vi "PID_controller_11.vi"() -> ()   [LabVIEW 2011]
uses:
  <vilib>/Platform/TimedLoop/XDataNode/timing_clust.ctl
  <vilib>/Platform/TimedLoop/XDataNode/nitl_modes.ctl
  <vilib>/Platform/TimedLoop/XDataNode/wakeup.ctl
  <vilib>/Platform/TimedLoop/XDataNode/XDataNode.xnode
  <vilib>/Platform/TimedLoop/XDataNode/XDNodeRunTimeDep.lvlib
panel:
  in  "stop 2":bool
  out "fit":cluster{"element":dbl, "Value":dbl}[](array[cluster])
  out "err_avg":dbl
  out "Setpoint":string
  out "Angle (deg)":string
  in  "Ks":dbl
  out "dt(s)":dbl
  out "windup error":dbl
  out "tPrev":dbl
  out "target value":dbl
  out "error(t-t0)":cluster{dbl, "Value":dbl}[](array[cluster])
  out "error":dbl
  out "tStart(s)":dbl
  out "S00":dbl
  out "S10":dbl
  out "S20":dbl
  out "S11":dbl
  out "S01":dbl
  out "weight":dbl[](array[numeric])
  in  "# of points to watch":i32
  in  "tSmooth(s)":dbl=-1.0
  out "t0":dbl
  out "error(t)":cluster{dbl, "Value":dbl}[](array[cluster])
  out "error out":errorcluster
  out "first":bool=TRUE
  out "P (torr)":string
  out "XY Graph":T1(graph)
  out "current value":dbl
  in  "Period (s)":dbl
  out "dValue":dbl
  out "derivative":dbl
  out "integral":dbl
  out "Current angle (deg)":dbl
  in  "Kd":dbl
  in  "Ki":dbl
  in  "Kp":dbl
  out "Current P (torr)":dbl
  in  "Set Point (torr)":dbl
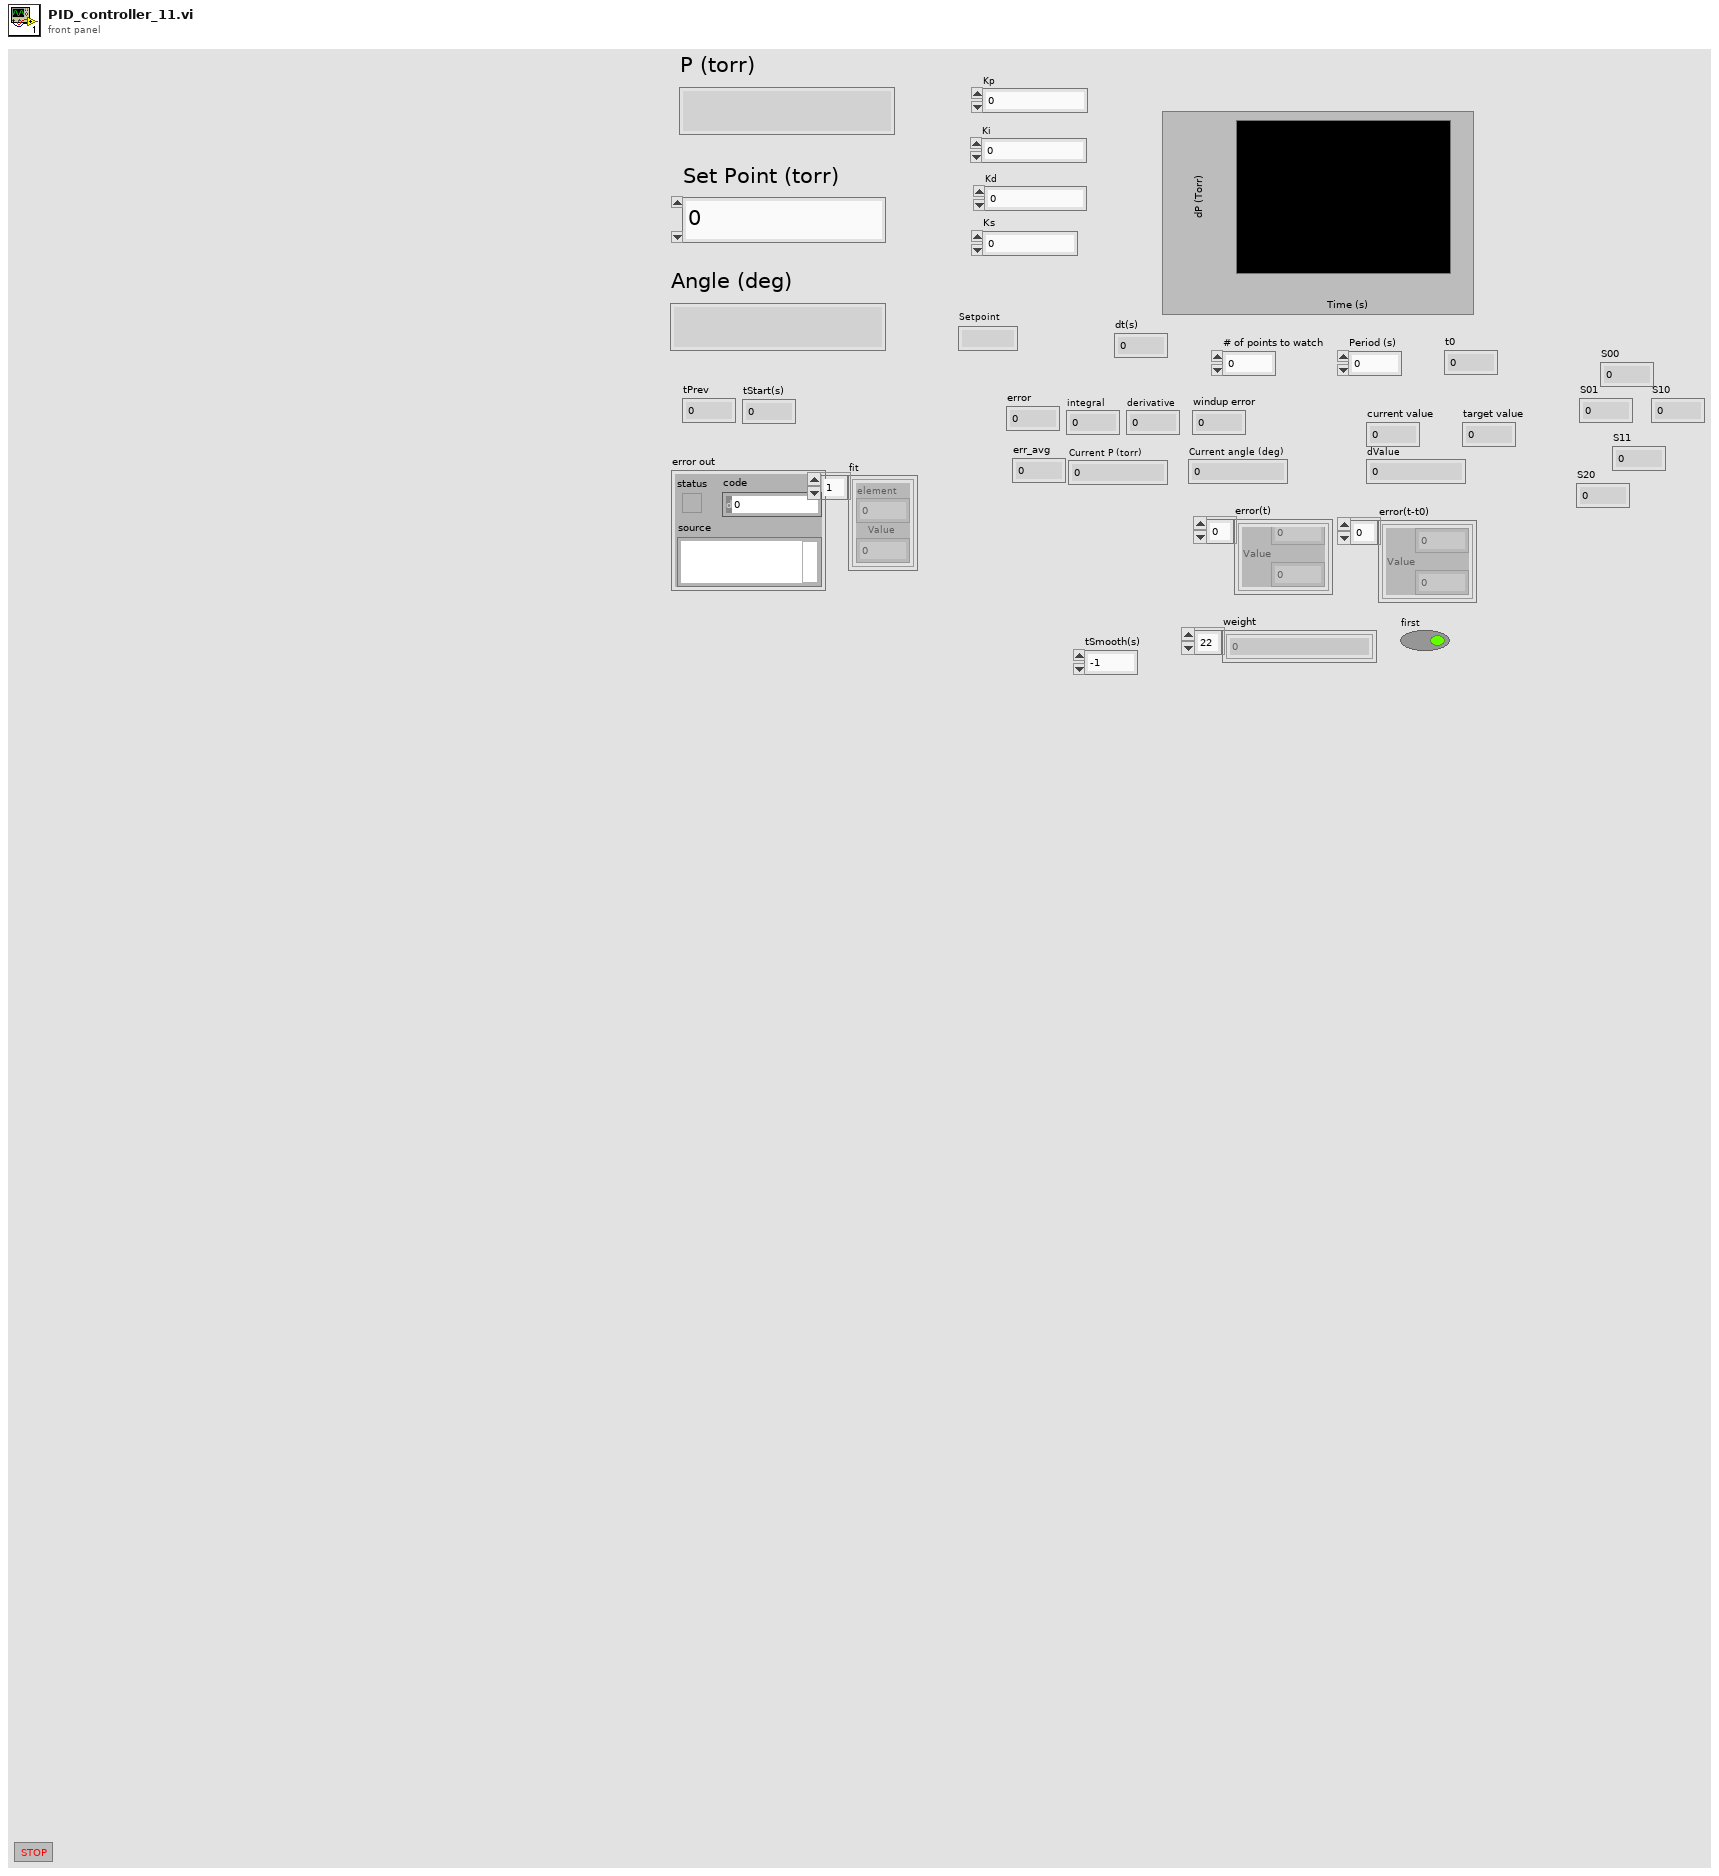
[diagram p1: front panel]
types:
  T1 = cluster{"Value":cluster{"element":dbl, "Value":dbl}[]}[]
  T2 = typedef "XDNodeRunTimeDep.lvlib/timing_clust.ctl" = cluster{"Expected End [f-1]":u64, "Actual End [f-1]":u64, "Finished Late? [f-1]":bool, "Expected End [i-1]":u64, "Actual End [i-1]":u64, "Finished Late? [i-1]":bool, "Expected Start [i]":u64, "Actual Start [i]":u64, "Expected Start [f]":u64, "Actual Start [f]":u64, "Source Name":string, "Structure Name":string, "Period":i64, "Deadline":i64, "Offset":i64, "Start":i64, "Priority":i32, "Timeout":i32, "Mode":T3, "Wakeup Reason":T4, "Error":errorcluster, "Source Type":string, "Secondary Source Type":string, "Global End Time":u64, "Global Start Time":u64, "Frame Duration":u64, "Iteration Duration":u64, "Assigned CPU":i32, "I/O Scan Engine Mode":u32}
  T3 = typedef "XDNodeRunTimeDep.lvlib/nitl_modes.ctl" = enum32{"No Change", "Process missed periods, maintain original phase", "Discard missed periods, maintain original phase", "Process missed periods, ignore original phase", "Discard missed periods, ignore original phase"}
  T4 = typedef "XDNodeRunTimeDep.lvlib/wakeup.ctl" = enum32{"Normal", "Aborted", "Asynchronous wakeup", "Timing source error", "Timed loop error", "Timeout"}
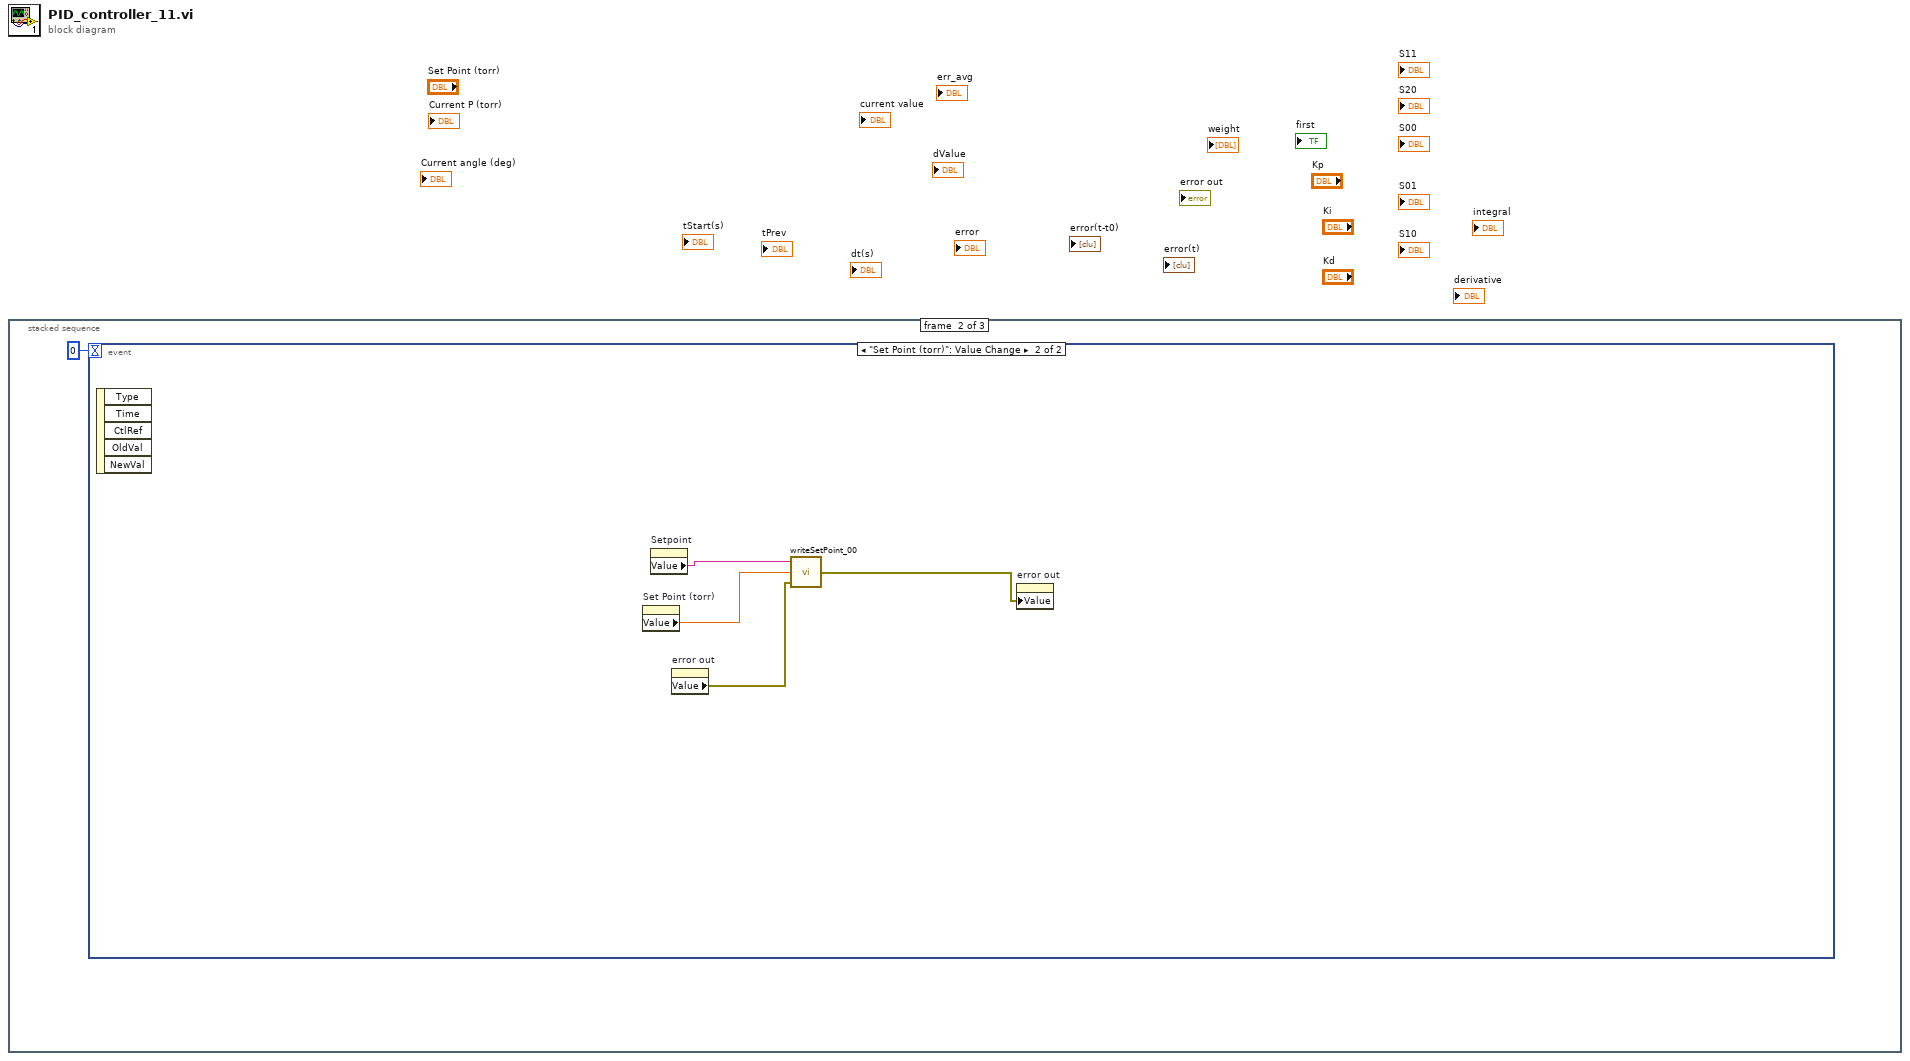
[diagram p0: block diagram]
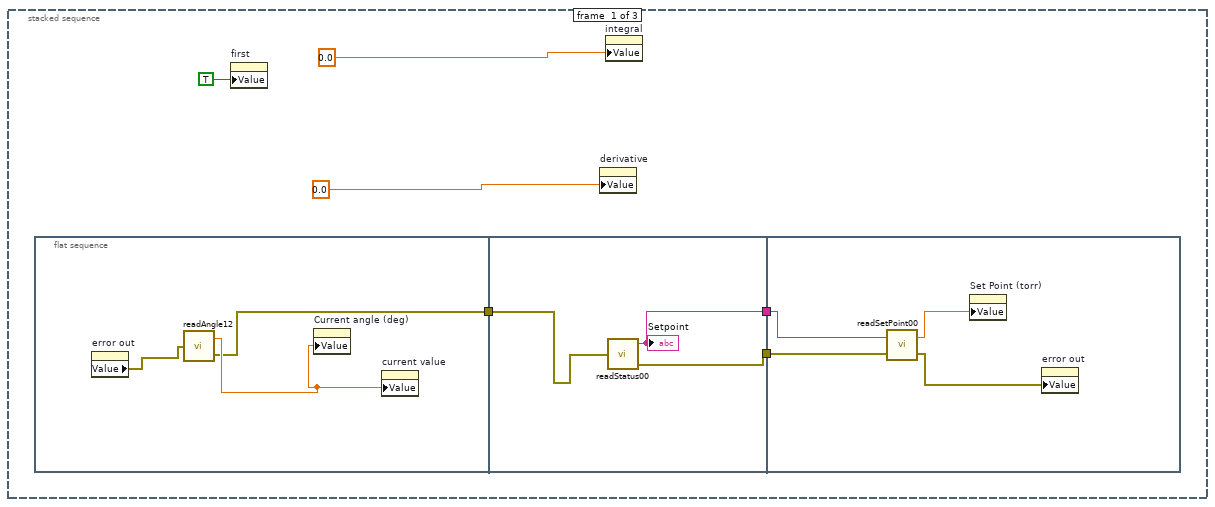
[diagram p2: hidden frame]
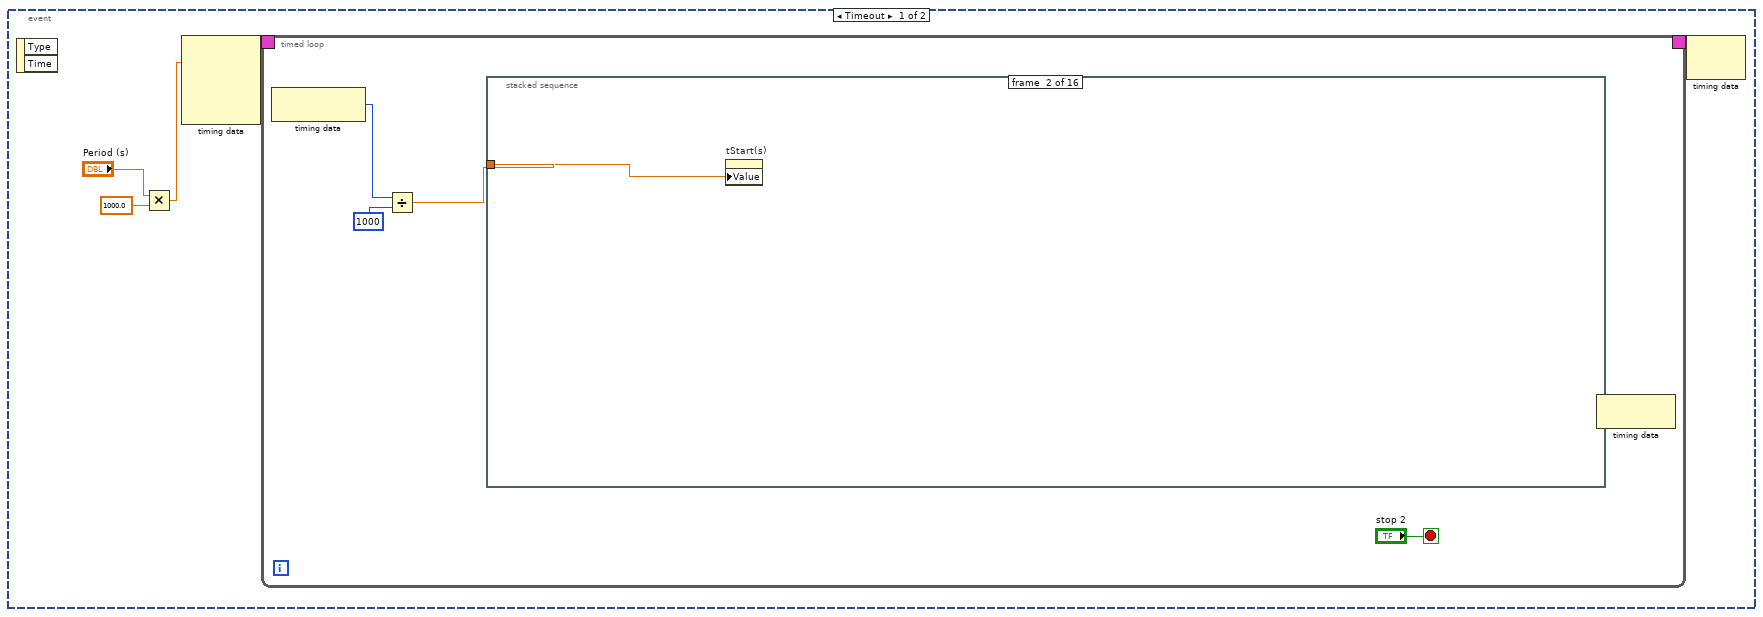
[diagram p3: hidden frame]
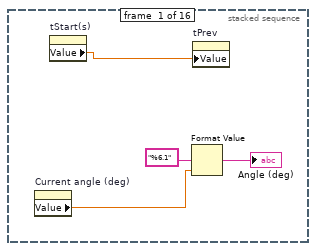
[diagram p4: hidden frame]
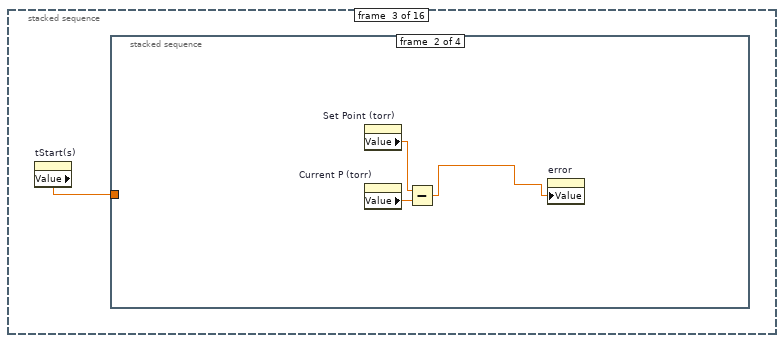
[diagram p5: hidden frame]
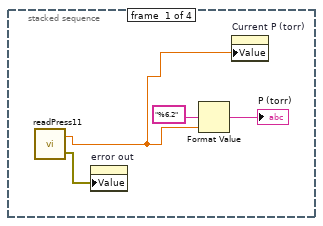
[diagram p6: hidden frame]
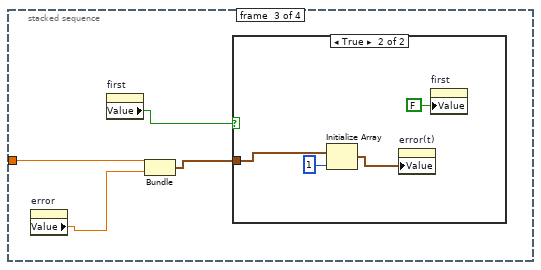
[diagram p7: hidden frame]
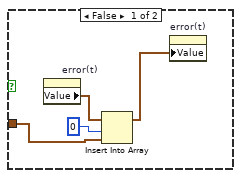
[diagram p8: hidden frame]
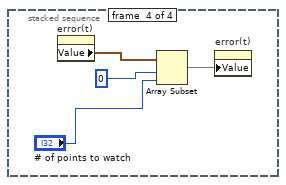
[diagram p9: hidden frame]
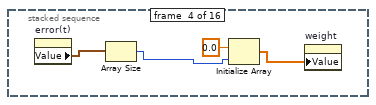
[diagram p10: hidden frame]
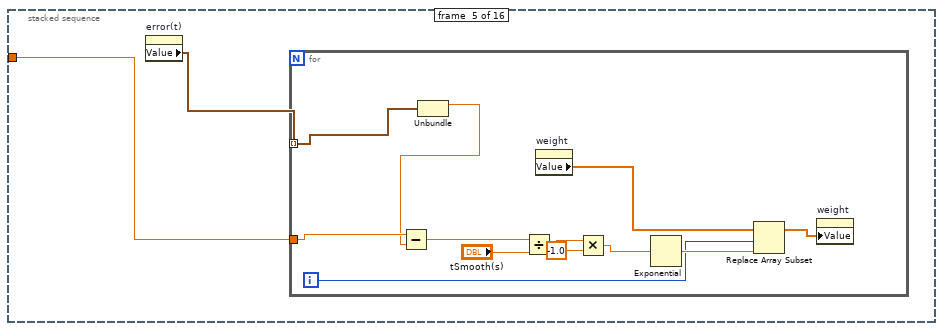
[diagram p11: hidden frame]
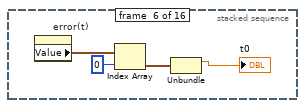
[diagram p12: hidden frame]
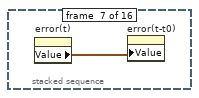
[diagram p13: hidden frame]
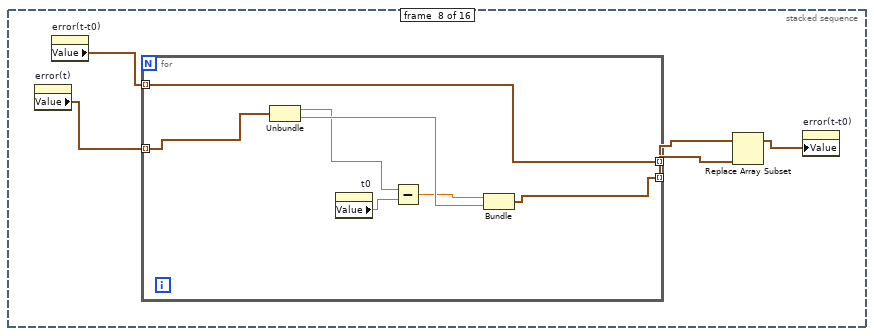
[diagram p14: hidden frame]
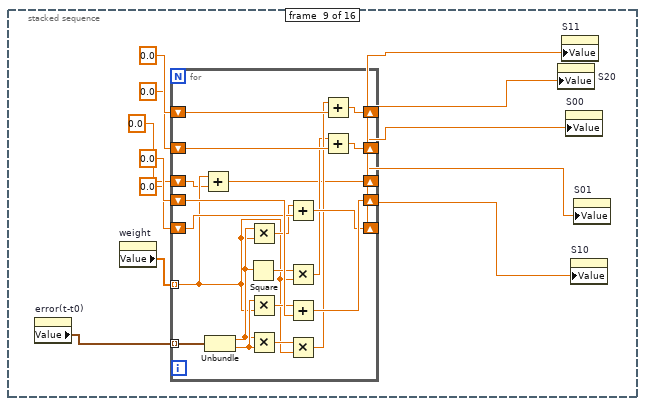
[diagram p15: hidden frame]
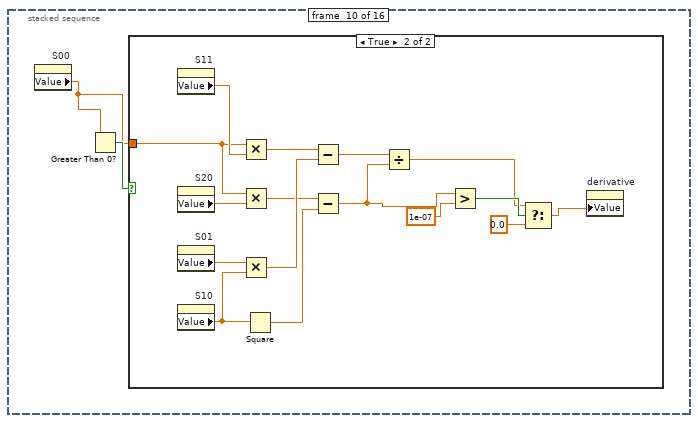
[diagram p16: hidden frame]
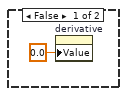
[diagram p17: hidden frame]
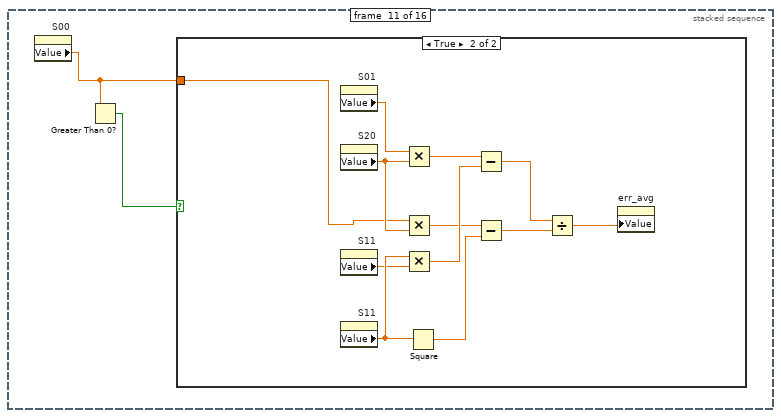
[diagram p18: hidden frame]
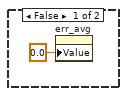
[diagram p19: hidden frame]
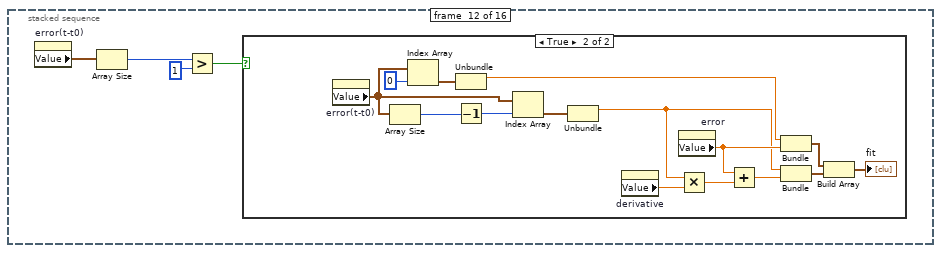
[diagram p20: hidden frame]
diagram:
  n1 = stacked-sequence {
    frame #0 {
      n2 = flat-sequence {
        tunnel: [w7] -> w1
        tunnel: [w12] -> w3
        tunnel: [w11] -> w2
        tunnel: w1 -> [w10]
        tunnel: w3 -> [w16]
        tunnel: w2 -> [w15]
        frame #0 {
          n3 = property on="error out" class="Clust (strict)"() -> ("Value"=w9:errorcluster)  [unwired: 2 in, 2 out]
          n4 = call "readAngle12.vi"("error in"=w9) -> ("angle"=w8:dbl, "error out"=w7:errorcluster)
          n5 = property on="Current angle (deg)" class="DigNum (strict)"("Value"=w8) -> ()  [unwired: 2 in, 2 out]
          n6 = property on="current value" class="DigNum (strict)"("Value"=w8) -> ()  [unwired: 2 in, 2 out]
        }
        frame #1 {
          n7 = call "readStatus00.vi"("error in"=w10) -> ("Setpoint"=w12:string, "error out"=w11:errorcluster)  [unwired: 1 out]
          "Setpoint" <- w12
        }
        frame #2 {
          n8 = call "readSetPoint00.vi"("error in"=w15, "Setpoint"=w16) -> ("error out"=w14:errorcluster, "P"=w13:dbl)
          n9 = property on="Set Point (torr)" class="DigNum (strict)"("Value"=w13) -> ()  [unwired: 2 in, 2 out]
          n10 = property on="error out" class="Clust (strict)"("Value"=w14) -> ()  [unwired: 2 in, 2 out]
        }
      }
      n11 = property on="first" class="Bool (strict)"("Value"=TRUE ("first")) -> ()  [unwired: 2 in, 2 out]
      n12 = property on="derivative" class="DigNum (strict)"("Value"=0.0 ("derivative")) -> ()  [unwired: 2 in, 2 out]
      n13 = property on="integral" class="DigNum (strict)"("Value"=0.0 ("integral")) -> ()  [unwired: 2 in, 2 out]
    }
    frame #1 {
      n14 = event shown="[1] \"Set Point (torr)\": Value Change" {
        selector: _ -> [_ _]
        dyn-events: _ -> [_ _]
        timeout: 0 -> [_ _]
        event Timeout {
          n15 = event-data() -> ()  [unwired: 1 in, 2 out]
          n16 = Multiply(x="Period (s)", y=1000.0) -> (x*y=w18:dbl)
          n17 = node-c288(w18) -> (w22:T2)  [unwired: 3 in]
          n18 = timed-loop {
            timing: w22 -> [_]
            timing-out: [_] -> w21
            stop <- "stop 2" stop-if-true
            n19 = node-c288() -> (w24:i64)  [unwired: 1 in]
            n20 = Divide(x=w24, y=i64 1000) -> (x/y=w23:dbl)
            n21 = stacked-sequence {
              tunnel: w23 -> [_ w31 _ _ w60 _ _ _ _ _ _ _ _ _ _ _]
              frame #0 {
                n22 = property on="Current angle (deg)" class="DigNum (strict)"() -> ("Value"=w27:dbl)  [unwired: 2 in, 2 out]
                n23 = property on="tStart(s)" class="DigNum (strict)"() -> ("Value"=w30:dbl)  [unwired: 2 in, 2 out]
                n24 = Format Value(format string="%6.1", value (0)=w27) -> (output string=→"Angle (deg)":string)  [unwired: 1 in]
                n25 = property on="tPrev" class="DigNum (strict)"("Value"=w30) -> ()  [unwired: 2 in, 2 out]
              }
              frame #1 {
                n26 = property on="tStart(s)" class="DigNum (strict)"("Value"=w31) -> ()  [unwired: 2 in, 2 out]
              }
              frame #2 {
                n27 = property on="tStart(s)" class="DigNum (strict)"() -> ("Value"=w32:dbl)  [unwired: 2 in, 2 out]
                n28 = stacked-sequence {
                  tunnel: w32 -> [_ _ w42 _]
                  frame #0 {
                    n29 = call "readPress11.vi"() -> ("P"=w34:dbl, "error out"=w33:errorcluster)  [unwired: 1 in]
                    n30 = property on="error out" class="Clust (strict)"("Value"=w33) -> ()  [unwired: 2 in, 2 out]
                    n31 = Format Value(format string="%6.2", value (0)=w34) -> (output string=→"P (torr)":string)  [unwired: 1 in]
                    n32 = property on="Current P (torr)" class="DigNum (strict)"("Value"=w34) -> ()  [unwired: 2 in, 2 out]
                  }
                  frame #1 {
                    n33 = property on="Set Point (torr)" class="DigNum (strict)"() -> ("Value"=w38:dbl)  [unwired: 2 in, 2 out]
                    n34 = property on="Current P (torr)" class="DigNum (strict)"() -> ("Value"=w39:dbl)  [unwired: 2 in, 2 out]
                    n35 = Subtract(x=w38, y=w39) -> (x-y=w37:dbl)
                    n36 = property on="error" class="DigNum (strict)"("Value"=w37) -> ()  [unwired: 2 in, 2 out]
                  }
                  frame #2 {
                    n37 = property on="error" class="DigNum (strict)"() -> ("Value"=w40:dbl)  [unwired: 2 in, 2 out]
                    n38 = property on="first" class="Bool (strict)"() -> ("Value"=w43:bool)  [unwired: 2 in, 2 out]
                    n39 = Bundle("Value"=w42, "Value"=w40) -> (w41:cluster{"Value":dbl, "Value":dbl})  [unwired: 1 in]
                    n40 = case shown="True" w43 {
                      tunnel: w41 -> [w45 w50]
                      frame False {
                        n41 = property on="error(t)" class="Arr (strict)"() -> ("Value"=w46:cluster{dbl, "Value":dbl}[])  [unwired: 2 in, 2 out]
                        n42 = Insert Into Array(array=w46, index=0, new element=w45) -> (w44:cluster{dbl, "Value":dbl}[])
                        n43 = property on="error(t)" class="Arr (strict)"("Value"=w44) -> ()  [unwired: 2 in, 2 out]
                      }
                      frame True {
                        n44 = Initialize Array(w50, 1 ("dimension size")) -> (w48:cluster{"Value":dbl, "Value":dbl}[])
                        n45 = property on="error(t)" class="Arr (strict)"("Value"=w48) -> ()  [unwired: 2 in, 2 out]
                        n46 = property on="first" class="Bool (strict)"("Value"=FALSE ("first")) -> ()  [unwired: 2 in, 2 out]
                      }
                    }
                  }
                  frame #3 {
                    n47 = property on="error(t)" class="Arr (strict)"() -> ("Value"=w53:cluster{dbl, "Value":dbl}[])  [unwired: 2 in, 2 out]
                    n48 = Array Subset(array=w53, index=0, length="# of points to watch") -> (w55:cluster{dbl, "Value":dbl}[])
                    n49 = property on="error(t)" class="Arr (strict)"("Value"=w55) -> ()  [unwired: 2 in, 2 out]
                  }
                }
              }
              frame #3 {
                n50 = property on="error(t)" class="Arr (strict)"() -> ("Value"=w59:cluster{dbl, "Value":dbl}[])  [unwired: 2 in, 2 out]
                n51 = Array Size(array=w59) -> (size(s)=w57:i32)
                n52 = Initialize Array(0.0 ("element"), w57) -> (w56:dbl[])
                n53 = property on="weight" class="Arr (strict)"("Value"=w56) -> ()  [unwired: 2 in, 2 out]
              }
              frame #4 {
                n54 = property on="error(t)" class="Arr (strict)"() -> ("Value"=w61:cluster{dbl, "Value":dbl}[])  [unwired: 2 in, 2 out]
                n55 = for {
                  tunnel: w61 -> [w73] mode=indexing
                  tunnel: w60 -> [w72]
                  i -> [w68]
                  n56 = Unbundle(w73) -> (w71:dbl)  [unwired: 1 out]
                  n57 = Subtract(x=w72, y=w71) -> (x-y=w66:dbl)
                  n58 = Divide(x=w66, y="tSmooth(s)") -> (x/y=w64:dbl)
                  n59 = property on="weight" class="Arr (strict)"() -> ("Value"=w69:dbl[])  [unwired: 2 in, 2 out]
                  n60 = Multiply(x=w64, y=-1.0) -> (x*y=w62:dbl)
                  n61 = Exponential(1:w62) -> (0:w70:dbl)
                  n62 = Replace Array Subset(array=w69, new element=w70, index=w68) -> (w67:dbl[])
                  n63 = property on="weight" class="Arr (strict)"("Value"=w67) -> ()  [unwired: 2 in, 2 out]
                }
              }
              frame #5 {
                n64 = property on="error(t)" class="Arr (strict)"() -> ("Value"=w77:cluster{dbl, "Value":dbl}[])  [unwired: 2 in, 2 out]
                n65 = Index Array(array=w77, index=0) -> (element=w75:cluster{dbl, "Value":dbl})
                n66 = Unbundle(w75) -> (→"t0":dbl)  [unwired: 1 out]
              }
              frame #6 {
                n67 = property on="error(t)" class="Arr (strict)"() -> ("Value"=w78:cluster{dbl, "Value":dbl}[])  [unwired: 2 in, 2 out]
                n68 = property on="error(t-t0)" class="Arr (strict)"("Value"=w78) -> ()  [unwired: 2 in, 2 out]
              }
              frame #7 {
                n69 = property on="error(t)" class="Arr (strict)"() -> ("Value"=w83:cluster{dbl, "Value":dbl}[])  [unwired: 2 in, 2 out]
                n70 = property on="error(t-t0)" class="Arr (strict)"() -> ("Value"=w81:cluster{dbl, "Value":dbl}[])  [unwired: 2 in, 2 out]
                n71 = for {
                  tunnel: w83 -> [w86] mode=indexing
                  tunnel: [w85] -> w82 mode=indexing
                  tunnel: w81 -> [w84] mode=indexing
                  tunnel: [w84] -> w80 mode=indexing
                  n72 = Unbundle(w86) -> (w87:dbl, "Value"=w89:dbl)
                  n73 = property on="t0" class="DigNum (strict)"() -> ("Value"=w90:dbl)  [unwired: 2 in, 2 out]
                  n74 = Subtract(x=w87, y=w90) -> (x-y=w88:dbl)
                  n75 = Bundle(w88, "Value"=w89) -> (w85:cluster{dbl, "Value":dbl})  [unwired: 1 in]
                }
                n76 = Replace Array Subset(array=w80, new element=w82) -> (w79:cluster{dbl, "Value":dbl}[])  [unwired: 1 in]
                n77 = property on="error(t-t0)" class="Arr (strict)"("Value"=w79) -> ()  [unwired: 2 in, 2 out]
              }
              frame #8 {
                n78 = property on="error(t-t0)" class="Arr (strict)"() -> ("Value"=w91:cluster{dbl, "Value":dbl}[])  [unwired: 2 in, 2 out]
                n79 = property on="weight" class="Arr (strict)"() -> ("Value"=w98:dbl[])  [unwired: 2 in, 2 out]
                n80 = for {
                  tunnel: w91 -> [w118] mode=indexing
                  shift-right: [w119] -> w93
                  shift-left: 0.0 -> [w122]
                  shift-right: [w115] -> w96
                  shift-left: 0.0 -> [w121]
                  shift-right: [w114] -> w95
                  shift-left: 0.0 -> [w120]
                  shift-right: [w116] -> w92
                  shift-left: 0.0 -> [w117]
                  tunnel: w98 -> [w105] mode=indexing
                  shift-right: [w103] -> w94
                  shift-left: 0.0 -> [w104]
                  n81 = Add(x=w105, y=w104) -> (x+y=w103:dbl)
                  n82 = Unbundle(w118) -> (w107:dbl, "Value"=w113:dbl)
                  n83 = Square(x=w107) -> (x^2=w109:dbl)
                  n84 = Multiply(x=w107, y=w105) -> (x*y=w106:dbl)
                  n85 = Multiply(x=w113, y=w105) -> (x*y=w112:dbl)
                  n86 = Multiply(x=w107, y=w113) -> (x*y=w111:dbl)
                  n87 = Add(x=w106, y=w117) -> (x+y=w116:dbl)
                  n88 = Multiply(x=w109, y=w105) -> (x*y=w108:dbl)
                  n89 = Add(x=w112, y=w122) -> (x+y=w119:dbl)
                  n90 = Multiply(x=w111, y=w105) -> (x*y=w110:dbl)
                  n91 = Add(x=w110, y=w121) -> (x+y=w115:dbl)
                  n92 = Add(x=w108, y=w120) -> (x+y=w114:dbl)
                }
                n93 = property on="S20" class="DigNum (strict)"("Value"=w95) -> ()  [unwired: 2 in, 2 out]
                n94 = property on="S11" class="DigNum (strict)"("Value"=w96) -> ()  [unwired: 2 in, 2 out]
                n95 = property on="S00" class="DigNum (strict)"("Value"=w94) -> ()  [unwired: 2 in, 2 out]
                n96 = property on="S10" class="DigNum (strict)"("Value"=w92) -> ()  [unwired: 2 in, 2 out]
                n97 = property on="S01" class="DigNum (strict)"("Value"=w93) -> ()  [unwired: 2 in, 2 out]
              }
              frame #9 {
                n98 = property on="S00" class="DigNum (strict)"() -> ("Value"=w123:dbl)  [unwired: 2 in, 2 out]
                n99 = Greater Than 0?(x=w123) -> (x > 0?=w124:bool)
                n100 = case shown="True" w124 {
                  tunnel: w123 -> [_ w133]
                  frame False {
                    n101 = property on="derivative" class="DigNum (strict)"("Value"=0.0 ("derivative")) -> ()  [unwired: 2 in, 2 out]
                  }
                  frame True {
                    n102 = property on="S11" class="DigNum (strict)"() -> ("Value"=w135:dbl)  [unwired: 2 in, 2 out]
                    n103 = property on="S20" class="DigNum (strict)"() -> ("Value"=w134:dbl)  [unwired: 2 in, 2 out]
                    n104 = property on="S01" class="DigNum (strict)"() -> ("Value"=w132:dbl)  [unwired: 2 in, 2 out]
                    n105 = property on="S10" class="DigNum (strict)"() -> ("Value"=w136:dbl)  [unwired: 2 in, 2 out]
                    n106 = Multiply(x=w133, y=w135) -> (x*y=w141:dbl)
                    n107 = Multiply(x=w133, y=w134) -> (x*y=w139:dbl)
                    n108 = Multiply(x=w132, y=w136) -> (x*y=w140:dbl)
                    n109 = Square(x=w136) -> (x^2=w138:dbl)
                    n110 = Subtract(x=w141, y=w140) -> (x-y=w137:dbl)
                    n111 = Subtract(x=w139, y=w138) -> (x-y=w131:dbl)
                    n112 = Divide(x=w137, y=w131) -> (x/y=w127:dbl)
                    n113 = Greater?(x=w131, y=1e-07) -> (0:w129:bool)
                    n114 = Select(t=w127, s=w129, f=0.0) -> (s? t:f=w128:dbl)
                    n115 = property on="derivative" class="DigNum (strict)"("Value"=w128) -> ()  [unwired: 2 in, 2 out]
                  }
                }
              }
              frame #10 {
                n116 = property on="S00" class="DigNum (strict)"() -> ("Value"=w142:dbl)  [unwired: 2 in, 2 out]
                n117 = Greater Than 0?(x=w142) -> (x > 0?=w143:bool)
                n118 = case shown="True" w143 {
                  tunnel: w142 -> [_ w146]
                  frame False {
                    n119 = property on="err_avg" class="DigNum (strict)"("Value"=0.0 ("Pavg")) -> ()  [unwired: 2 in, 2 out]
                  }
                  frame True {
                    n120 = property on="S01" class="DigNum (strict)"() -> ("Value"=w147:dbl)  [unwired: 2 in, 2 out]
                    n121 = property on="S20" class="DigNum (strict)"() -> ("Value"=w150:dbl)  [unwired: 2 in, 2 out]
                    n122 = property on="S11" class="DigNum (strict)"() -> ("Value"=w148:dbl)  [unwired: 2 in, 2 out]
                    n123 = property on="S11" class="DigNum (strict)"() -> ("Value"=w149:dbl)  [unwired: 2 in, 2 out]
                    n124 = Multiply(x=w147, y=w150) -> (x*y=w155:dbl)
                    n125 = Multiply(x=w146, y=w150) -> (x*y=w152:dbl)
                    n126 = Multiply(x=w149, y=w148) -> (x*y=w156:dbl)
                    n127 = Square(x=w149) -> (x^2=w153:dbl)
                    n128 = Subtract(x=w155, y=w156) -> (x-y=w151:dbl)
                    n129 = Subtract(x=w152, y=w153) -> (x-y=w154:dbl)
                    n130 = Divide(x=w151, y=w154) -> (x/y=w145:dbl)
                    n131 = property on="err_avg" class="DigNum (strict)"("Value"=w145) -> ()  [unwired: 2 in, 2 out]
                  }
                }
              }
              frame #11 {
                n132 = property on="error(t-t0)" class="Arr (strict)"() -> ("Value"=w160:cluster{dbl, "Value":dbl}[])  [unwired: 2 in, 2 out]
                n133 = Array Size(array=w160) -> (size(s)=w159:i32)
                n134 = Greater?(x=w159, y=1) -> (0:w157:bool)
                n135 = case shown="True" w157 {
                  frame False {
                  }
                  frame True {
                    n136 = property on="error(t-t0)" class="Arr (strict)"() -> ("Value"=w164:cluster{dbl, "Value":dbl}[])  [unwired: 2 in, 2 out]
                    n137 = Array Size(array=w164) -> (size(s)=w174:i32)
                    n138 = Index Array(array=w164, index=0) -> (element=w172:cluster{dbl, "Value":dbl})
                    n139 = Unbundle(w172) -> (w167:dbl)  [unwired: 1 out]
                    n140 = Decrement(x=w174) -> (x-1=w173:i32)
                    n141 = Index Array(array=w164, index=w173) -> (element=w171:cluster{dbl, "Value":dbl})
                    n142 = Unbundle(w171) -> (w165:dbl)  [unwired: 1 out]
                    n143 = property on="derivative" class="DigNum (strict)"() -> ("Value"=w170:dbl)  [unwired: 2 in, 2 out]
                    n144 = property on="error" class="DigNum (strict)"() -> ("Value"=w168:dbl)  [unwired: 2 in, 2 out]
                    n145 = Multiply(x=w165, y=w170) -> (x*y=w169:dbl)
                    n146 = Add(x=w168, y=w169) -> (x+y=w166:dbl)
                    n147 = Bundle(w167, "Value"=w168) -> (w163:cluster{dbl, "Value":dbl})  [unwired: 1 in]
                    n148 = Bundle(w165, w166) -> (w162:cluster{dbl, dbl})  [unwired: 1 in]
                    n149 = Build Array(w163, w162) -> (→"fit":cluster{dbl, "Value":dbl}[])
                  }
                }
              }
              frame #12 {
                n150 = property on="error" class="DigNum (strict)"() -> ("Value"=w180:dbl)  [unwired: 2 in, 2 out]
                n151 = property on="tPrev" class="DigNum (strict)"() -> ("Value"=w181:dbl)  [unwired: 2 in, 2 out]
                n152 = property on="tStart(s)" class="DigNum (strict)"() -> ("Value"=w182:dbl)  [unwired: 2 in, 2 out]
                n153 = Subtract(x=w182, y=w181) -> (x-y=w176:dbl)
                n154 = property on="dt(s)" class="DigNum (strict)"("Value"=w176) -> ()  [unwired: 2 in, 2 out]
                n155 = property on="integral" class="DigNum (strict)"() -> ("Value"=w178:dbl)  [unwired: 2 in, 2 out]
                n156 = Multiply(x=w180, y=w176) -> (x*y=w179:dbl)
                n157 = Add(x=w179, y=w178) -> (x+y=w177:dbl)
                n158 = property on="integral" class="DigNum (strict)"("Value"=w177) -> ()  [unwired: 2 in, 2 out]
              }
              frame #13 {
                n159 = property on="error" class="DigNum (strict)"() -> ("Value"=w183:dbl)  [unwired: 2 in, 2 out]
                n160 = property on="Kp" class="DigNum (strict)"() -> ("Value"=w193:dbl)  [unwired: 2 in, 2 out]
                n161 = property on="integral" class="DigNum (strict)"() -> ("Value"=w191:dbl)  [unwired: 2 in, 2 out]
                n162 = property on="derivative" class="DigNum (strict)"() -> ("Value"=w189:dbl)  [unwired: 2 in, 2 out]
                n163 = property on="Ki" class="DigNum (strict)"() -> ("Value"=w192:dbl)  [unwired: 2 in, 2 out]
                n164 = property on="Kd" class="DigNum (strict)"() -> ("Value"=w190:dbl)  [unwired: 2 in, 2 out]
                n165 = Multiply(x=w190, y=w189) -> (x*y=w186:dbl)
                n166 = Multiply(x=w192, y=w191) -> (x*y=w187:dbl)
                n167 = Multiply(x=w193, y=w183) -> (x*y=w188:dbl)
                n168 = Add(x=w188, y=w187) -> (x+y=w185:dbl)
                n169 = Add(x=w185, y=w186) -> (x+y=w184:dbl)
                n170 = property on="dValue" class="DigNum (strict)"("Value"=w184) -> ()  [unwired: 2 in, 2 out]
              }
              frame #14 {
                w203 = 90.0 ("y")
                n171 = property on="dValue" class="DigNum (strict)"() -> ("Value"=w210:dbl)  [unwired: 2 in, 2 out]
                n172 = property on="current value" class="DigNum (strict)"() -> ("Value"=w211:dbl)  [unwired: 2 in, 2 out]
                n173 = Add(x=w211, y=w210) -> (x+y=w194:dbl)
                "target value" <- w194
                n174 = Less Than 0?(x=w194) -> (x < 0?=w207:bool)
                n175 = Select(t=0.0, s=w207, f=w194) -> (s? t:f=w204:dbl)
                n176 = property on="error out" class="Clust (strict)"() -> ("Value"=w209:errorcluster)  [unwired: 2 in, 2 out]
                n177 = Greater?(x=w204, y=w203) -> (0:w205:bool)
                n178 = Select(t=w203, s=w205, f=w204) -> (s? t:f=w195:dbl)
                n179 = Subtract(x=w195, y=w194) -> (x-y=w202:dbl)
                "windup error" <- w202
                n180 = call "setAngle_00.vi"("error in (no error)"=w209, "Angle (deg)"=w195) -> ("error out"=w208:errorcluster)
                n181 = property on="Current angle (deg)" class="DigNum (strict)"("Value"=w195) -> ()  [unwired: 2 in, 2 out]
                n182 = property on="dt(s)" class="DigNum (strict)"() -> ("Value"=w201:dbl)  [unwired: 2 in, 2 out]
                n183 = property on="current value" class="DigNum (strict)"("Value"=w195) -> ()  [unwired: 2 in, 2 out]
                n184 = property on="error out" class="Clust (strict)"("Value"=w208) -> ()  [unwired: 2 in, 2 out]
                n185 = Multiply(x=w202, y=w201) -> (x*y=w200:dbl)
                n186 = property on="integral" class="DigNum (strict)"() -> ("Value"=w197:dbl)  [unwired: 2 in, 2 out]
                n187 = Multiply(x="Ks", y=w200) -> (x*y=w198:dbl)
                n188 = Add(x=w198, y=w197) -> (x+y=w196:dbl)
                n189 = property on="integral" class="DigNum (strict)"("Value"=w196) -> ()  [unwired: 2 in, 2 out]
              }
              frame #15 {
                n190 = property on="fit" class="Arr (strict)"() -> ("Value"=w214:cluster{"element":dbl, "Value":dbl}[])  [unwired: 2 in, 2 out]
                n191 = property on="error(t-t0)" class="Arr (strict)"() -> ("Value"=w213:cluster{dbl, "Value":dbl}[])  [unwired: 2 in, 2 out]
                n192 = Build Cluster Array(w213, w214) -> (→"XY Graph":T1)
              }
            }
            n193 = node-c288() -> ()  [unwired: 1 in, 1 out]
          }
          n194 = node-c288(w21) -> ()  [unwired: 1 out]
        }
        event "Set Point (torr)": Value Change {
          n195 = event-data() -> ()  [unwired: 1 in, 5 out]
          n196 = property on="Set Point (torr)" class="DigNum (strict)"() -> ("Value"=w224:dbl)  [unwired: 2 in, 2 out]
          n197 = property on="Setpoint" class="Str"() -> ("Value"=w225:string)  [unwired: 2 in, 2 out]
          n198 = property on="error out" class="Clust (strict)"() -> ("Value"=w223:errorcluster)  [unwired: 2 in, 2 out]
          n199 = call "writeSetPoint_00.vi"("error in"=w223, "P (Torr)"=w224, "Setpoint"=w225) -> ("error out"=w222:errorcluster)
          n200 = property on="error out" class="Clust (strict)"("Value"=w222) -> ()  [unwired: 2 in, 2 out]
        }
      }
    }
    frame #2 {
      n201 = flat-sequence {
        frame #0 {
          n202 = call "WriteAdaptorr03.vi"("string to write"="D5") -> ()  [unwired: 1 in, 1 out]
        }
        frame #1 {
          n203 = property on="Setpoint" class="Str"() -> ("Value"=w228:string)  [unwired: 2 in, 2 out]
          n204 = Concatenate Strings("Press ", w228, " on AdapTorr") -> (w227:string)
          n205 = One Button Dialog(message=w227) -> ()  [unwired: 1 in, 1 out]
        }
      }
    }
  }
